vi "rs3_CropRGB.vi"(4 "Output Width X":i32, 5 "Output Height Y":i32, 6 "Start X":i32, 7 "start Y":i32, 8 "Zoom":bool=TRUE, 9 "Input Width X":i32=848, 10 "Input Height Y":i32=480, 11 "RGB Array":u8[](array[numeric])=array[1221120 elements]) -> (3 "New RGB Array":u8[](array[numeric]))   [LabVIEW 2017, in "libRealSense3.lvlib"]
uses:
  libRealSense3.lvlib
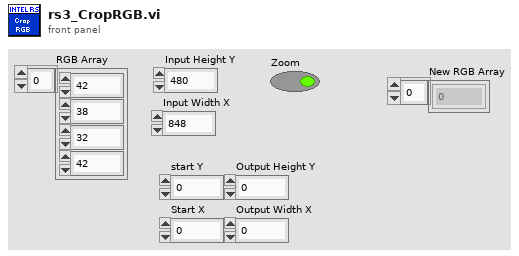
[diagram p1: front panel]
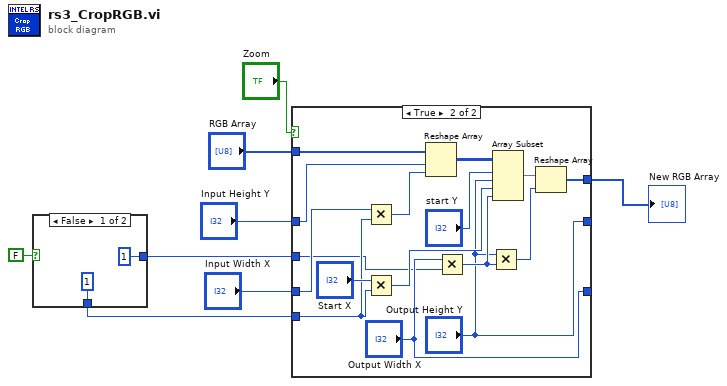
[diagram p0: block diagram]
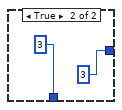
[diagram p2: hidden frame]
diagram:
  n1 = case shown="False" FALSE {
    tunnel: [1 ("y") 3 ("y")] -> w3
    tunnel: [1 ("y") 3 ("y")] -> w2
    frame False {
    }
    frame True {
    }
  }
  n2 = case shown="True" "Zoom" {
    tunnel: "RGB Array" -> [w15 w28]
    tunnel: "Input Height Y" -> [w14 w27]
    tunnel: [w15 w25] -> w6
    tunnel: "Input Width X" -> [w13 w24]
    tunnel: [w14 "Output Height Y"] -> _
    tunnel: [w13 "Output Width X"] -> _
    tunnel: w3 -> [_ w17]
    tunnel: w2 -> [_ w16]
    frame False {
    }
    frame True {
      n3 = Multiply(x=w24, y=w17) -> (x*y=w23:i32)
      n4 = Multiply(x="Start X", y=w17) -> (x*y=w21:i32)
      n5 = Reshape Array(w28, w27, w23) -> (w26:u8[][])
      n6 = Multiply(x="Output Width X", y=w16) -> (x*y=w20:i32)
      n7 = Multiply(x="Output Height Y", y=w20) -> (x*y=w29:i32)
      n8 = Array Subset(array=w26, index (row)="start Y", length (row)="Output Height Y", index (col)=w21, length (col)=w20) -> (w30:u8[][])
      n9 = Reshape Array(w30, w29) -> (w25:u8[])
    }
  }
  "New RGB Array" <- w6
